vi "_Copy 1.vi"(0 "XRef":T5, 1 "State In":T1) -> (14 "Reply":T3, 15 "Fatal Error Out":T2, 16 "State Out":T1)   [LabVIEW 2014, in "Browse_NEVSTOP-LAB.xnode"]
uses:
  <userlib>/_NEVSTOP/Browse_NEVSTOP-LAB.xnode
  <vilib>/XNodeSupport/XNodeXNodeRef.ctl
  <userlib>/_NEVSTOP/_xnode_browse_nevstoplab_support/_State 1.ctl
  <vilib>/XNodeSupport/XNodeStringArray.ctl
  <vilib>/XNodeSupport/XNodeString.ctl
  <vilib>/XNodeSupport/XNodeErrorCluster.ctl
  <vilib>/XNodeSupport/NI_XNodeSupport.lvlib
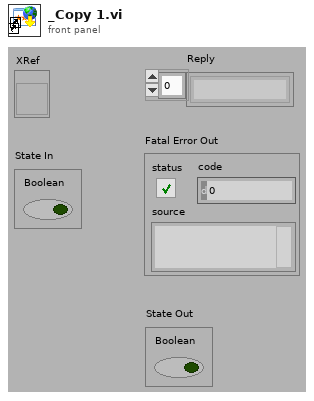
[diagram p1: front panel]
types:
  T1 = typedef "Browse_NEVSTOP-LAB.xnode/_State 1.ctl" = cluster{"Boolean":bool}
  T2 = typedef "NI_XNodeSupport.lvlib/XNodeErrorCluster.ctl" = errorcluster
  T3 = typedef "NI_XNodeSupport.lvlib/XNodeStringArray.ctl" = T4[]
  T4 = typedef "NI_XNodeSupport.lvlib/XNodeString.ctl" = string
  T5 = typedef "NI_XNodeSupport.lvlib/XNodeXNodeRef.ctl" = refnum<vi>
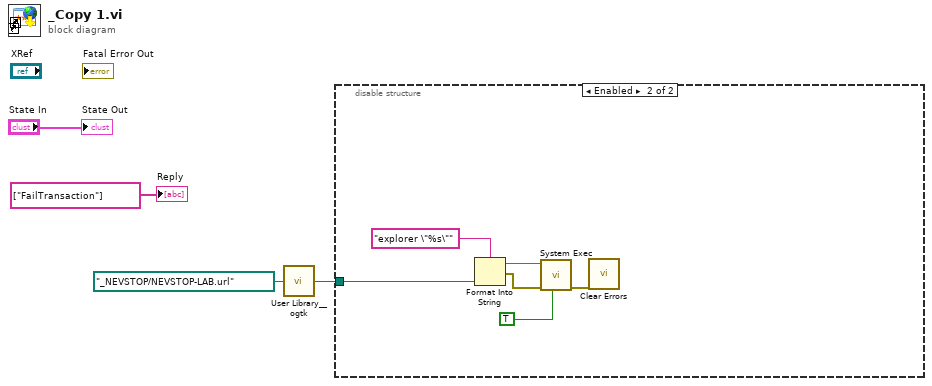
[diagram p0: block diagram]
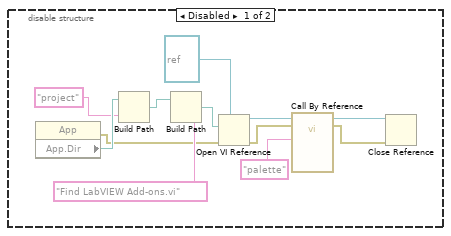
[diagram p2: hidden frame]
diagram:
  n1 = call <userlib>:"User Library__ogtk.vi"("Relative path (.)"=path "_NEVSTOP/NEVSTOP-LAB.url") -> ("User Library (+ Relative)"=w1:path)
  n2 = disable-structure shown="Enabled" {
    disable-tunnel: w1 -> [_ w22]
    frame Disabled {
      n3 = property class="App"() -> (error out=w11:errorcluster, "App.Dir"=w16:path)  [unwired: 2 in, 1 out]
      n4 = Build Path(base path=w16, name or relative path="project") -> (appended path=w14:path)
      n5 = Build Path(base path=w14, name or relative path="Find LabVIEW Add-ons.vi") -> (appended path=w12:path)
      n6 = Open VI Reference(type specifier VI Refnum (for type only)=refnum<vi> refnum ("reference"), vi path=w12, error in (no error)=w11) -> (vi reference=w9:refnum<vi>, error out=w6:errorcluster)  [unwired: 3 in]
      n7 = call-by-ref "?"(reference=w9, error in=w6, "Source"="palette") -> (reference out=w5:refnum<vi>, error out=w7:errorcluster)  [unwired: 11 in]
      n8 = Close Reference(reference=w5, error in (no error)=w7) -> ()  [unwired: 1 out]
    }
    frame Enabled {
      n9 = Format Into String(format string="explorer \"%s\"" ("command line"), w22) -> (resulting string=w20:string, error out=w17:errorcluster)  [unwired: 2 in]
      n10 = call <vilib>:"System Exec.vi"("run minimized? (F)"=TRUE, "error in (no error)"=w17, "command line"=w20) -> ("error out"=w18:errorcluster)  [unwired: 5 in, 3 out]
      n11 = call <vilib>:"Clear Errors.vi"("error in (no error)"=w18) -> ()  [unwired: 5 in, 2 out]
    }
  }
  "Reply" <- T3 ["FailTransaction"] ("Reply")
  "State Out" <- "State In"
